vi "Configure Device.vi"(8 "error in":errorcluster, 11 "PPT in":refnum<class "PPT.lvclass">) -> (0 "error out":errorcluster, 3 "PPT out":refnum<class "PPT.lvclass">, 4 "SP":dbl, 5 "Settable?":bool)   [LabVIEW 2018, in "PPT Library.lvlib" / "PPT.lvclass"]
uses:
  PPT.lvclass
  reusable/Session APIs/Serial/Serial Session.lvclass
  <vilib>/Utility/config.llb/NI_LVConfig.lvlib
  <vilib>/Utility/config.llb/Read Key (String).vi
  <vilib>/Utility/config.llb/Read Key (U32).vi
  reusable/Session APIs/File Access/Config Data/Config Data.lvclass
  reusable/Session APIs/Session Log/System Log.lvclass
  Configurable Device/Configurable Device.lvclass
  <vilib>/ErrorRing/Error Ring.xnode
  C:/Program Files (x86)/National Instruments/LabVIEW 2018/user.lib/_Session Fwk/Session - Root.lvclass
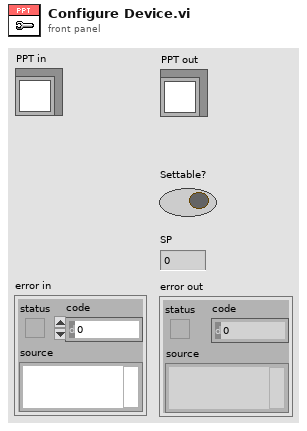
[diagram p1: front panel]
types:
  T1 = enum16{"atm", "bar", "cmwc", "ftwc", "inhg", "inwc", "kgcm", "kpa", "mbar", "mmhg", "mpa", "mwc", "psi", "user", "lcom", "pfs"}
  T2 = typedef "Serial Session.lvclass/Session Handle.ctl" = refnum<data-value>
  T3 = typedef "Config Data.lvclass/Config Session.ctl" = refnum<data-value>
  T4 = typedef "NI_LVConfig.lvlib/Config Data RefNum.ctl" = refnum<k1>
  T5 = typedef "Session - Root.lvclass/Session Handle.ctl" = refnum<data-value>
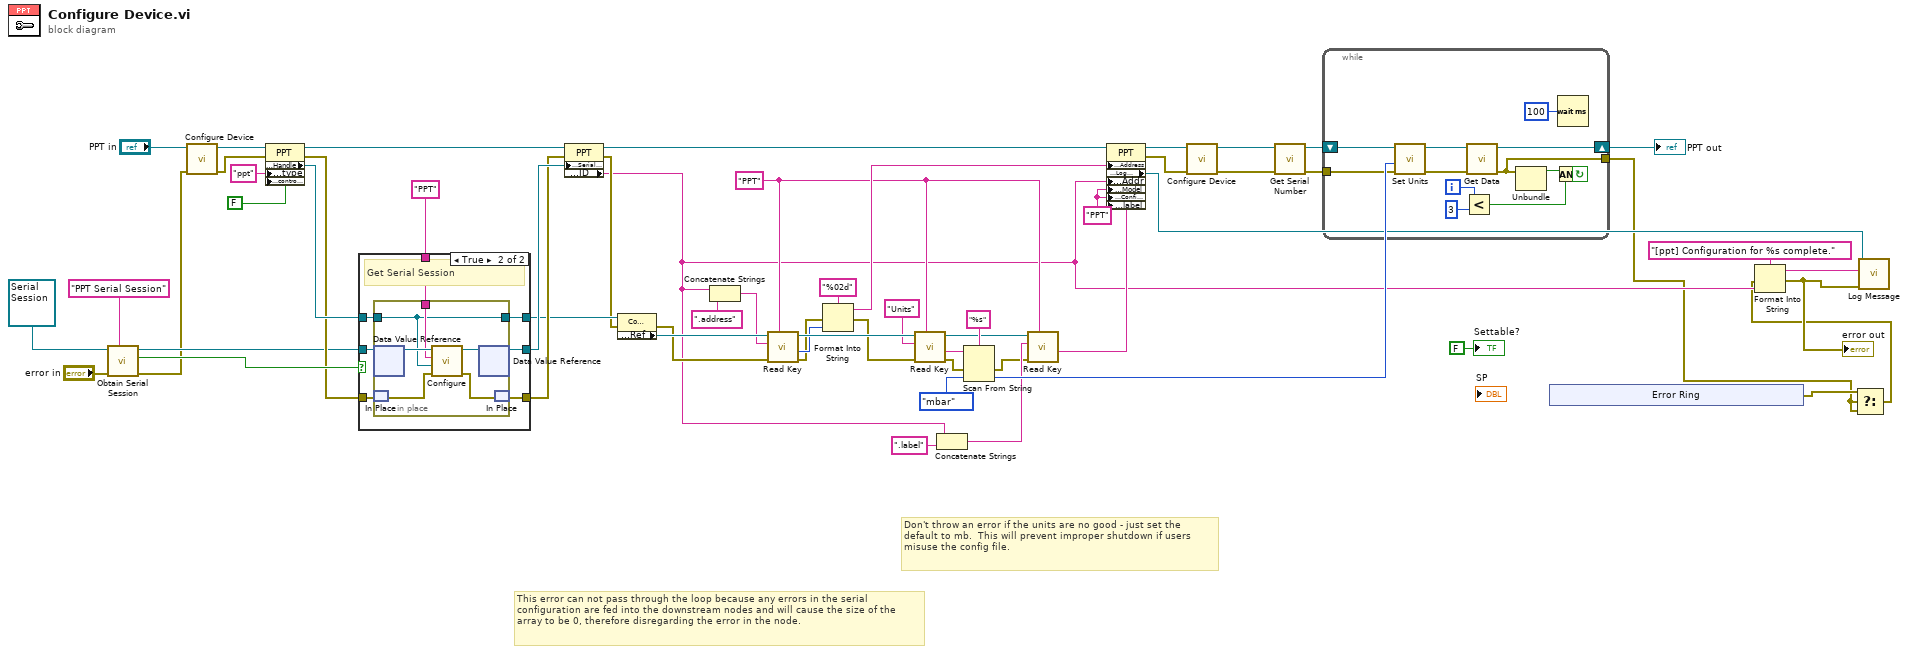
[diagram p0: block diagram]
diagram:
  w5 = "PPT" ("Model")
  w14 = "PPT" ("section")
  # "This error can not pass through the loop because any errors in the serial configuration are fed into the downstream nodes and will cause the size of the array to be 0, therefore disregarding the error in the node."
  # "Don't throw an error if the units are no good - just set the default to mb.  This will prevent improper shutdown if users misuse the config file."
  n1 = call "Obtain Serial Session.vi"("Session Name ()"="PPT Serial Session", "error in"="error in", "Serial Session in"=refnum<class "Serial Session.lvclass"> refnum) -> ("error out"=w19:errorcluster, "created new?"=w61:bool, "hSerial"=w57:T2)  [unwired: 6 in]
  n2 = call-parent "Configure Device.vi"("error in"=w19, "Device in"="PPT in") -> ("error out"=w18:errorcluster, "Device out"=w20:refnum<class "PPT.lvclass">)  [unwired: 6 in, 2 out]
  n3 = property class="PPT"(reference=w20, error in=w18, "Accessors:type"="ppt" ("type"), "Accessors:controller_"=FALSE ("controller_")) -> (reference out=w53:refnum<class "PPT.lvclass">, error out=w59:errorcluster, "Accessors:Handle"=w60:T3)
  n4 = case shown="True" w61 {
    tunnel: w57 -> [w64 w71]
    tunnel: w59 -> [w63 w67]
    tunnel: [w64 w70] -> w52
    tunnel: [w63 w69] -> w51
    tunnel: w60 -> [w62 w68]
    tunnel: [w62 w66] -> w42
    tunnel: "PPT" ("section") -> [_ w65]
    frame False {
    }
    frame True {
      # "Get Serial Session"
      n5 = in-place {
        in-place-border: w68 -> [w72]
        in-place-border: w65 -> [w73]
        in-place-border: [w72] -> w66
        n6 = in-place-dvr #1(w71) -> (w77:refnum<class "Serial Session.lvclass">)  [unwired: 1 out]
        n7 = in-place-match #2(w67) -> (w76:errorcluster)
        n8 = call "Configure.vi"("error in"=w76, "Config Handle"=w72, "section"=w73, "Serial Session in"=w77) -> ("error out"=w75:errorcluster, "Serial Session out"=w74:refnum<class "Serial Session.lvclass">)  [unwired: 6 in]
        n9 = in-place-dvr #1(w74) -> (w70:T2)  [unwired: 1 out]
        n10 = in-place-match #2(w75) -> (w69:errorcluster)
      }
    }
  }
  n11 = property class="PPT"(reference=w53, error in=w51, "Accessors:Serial Session"=w52) -> (reference out=w48:refnum<class "PPT.lvclass">, error out=w41:errorcluster, "Accessors:ID"=w10:string)
  n12 = property class="Config Data"(reference=w42, error in=w41) -> (error out=w29:errorcluster, "Accessors:Ref"=w40:T4)  [unwired: 1 out]
  n13 = Concatenate Strings(w10, ".address" ("string")) -> (w13:string)
  n14 = call-poly <vilib>:"Read Key.vi"("section"=w14, "error in (no error)"=w29, "key"=w13, "refnum"=w40) -> ("error out"=w28:errorcluster, "value"=w38:u32, "refnum out"=w50:T4)  [unwired: 4 in, 1 out]
  n15 = Format Into String(format string="%02d", error in=w28, w38) -> (resulting string=w47:string, error out=w27:errorcluster)  [unwired: 1 in]
  n16 = call-poly <vilib>:"Read Key.vi"("section"=w14, "error in (no error)"=w27, "key"="Units", "refnum"=w50) -> ("error out"=w33:errorcluster, "value"=w46:string, "refnum out"=w15:T4)  [unwired: 4 in, 1 out]
  n17 = Concatenate Strings(w10, ".label" ("string")) -> (w16:string)
  n18 = Scan From String(format string="%s", input string=w46, error in=w33, default 1=T1."mbar" ("units")) -> (error out=w11:errorcluster, output 1=w43:T1)  [unwired: 1 in, 2 out]
  n19 = call-poly <vilib>:"Read Key.vi"("section"=w14, "error in (no error)"=w11, "key"=w16, "refnum"=w15) -> ("value"=w12:string)  [unwired: 4 in, 3 out]
  n20 = property class="PPT"(reference=w48, "Accessors:Address"=w47, "Accessors:Addr"=w10, "Accessors:Model"=w5, "Accessors:Config Section"=w5, "Accessors:label"=w12) -> (reference out=w4:refnum<class "PPT.lvclass">, error out=w2:errorcluster, "Accessors:Log Session"=w36:T5)  [unwired: 1 in]
  n21 = call-parent "Configure Device.vi"("error in"=w2, "Device in"=w4) -> ("error out"=w1:errorcluster, "Device out"=w3:refnum<class "PPT.lvclass">)  [unwired: 6 in, 2 out]
  n22 = call "Get Serial Number.vi"("error in"=w1, "PPT in"=w3) -> ("error out"=w24:errorcluster, "PPT out"=w25:refnum<class "PPT.lvclass">)  [unwired: 7 in, 1 out]
  n23 = call "Set Units.vi"("error in"=w24, "units"=w43, "PPT in"=w25) -> ("error out"=w30:errorcluster, "PPT out"=w32:refnum<class "PPT.lvclass">)  [unwired: 7 in]
  n24 = while {
    shift-right: [w86] -> w31
    shift-left: w32 -> [w87]
    tunnel: [w80] -> w7
    tunnel: w30 -> [w79]
    i -> [w84]
    stop <- w81 continue-if-true
    n25 = Less?(x=w84, y=3) -> (x < y?=w82:bool)
    n26 = call-dynamic "Get Data.vi"("error in"=w79, "PPT in"=w87) -> ("error out"=w80:errorcluster, "PPT out"=w86:refnum<class "PPT.lvclass">)  [unwired: 7 in, 1 out]
    n27 = Unbundle(w80) -> ("status"=w85:bool)  [unwired: 2 out]
    n28 = And(x=w85, y=w82) -> (x .and. y?=w81:bool)
    n29 = Wait (ms)(milliseconds to wait=u32 100) -> ()  [unwired: 1 out]
  }
  "PPT out" <- w31
  n30 = xnode "Error Ring"() -> ("error out"=w8:errorcluster)
  n31 = Select(t=w8, s=w7, f=w7) -> (s? t:f=w6:errorcluster)
  n32 = Format Into String(format string="[ppt] Configuration for %s complete.", error in=w6, w10) -> (resulting string=w34:string, error out=w9:errorcluster)  [unwired: 1 in]
  "error out" <- w9
  n33 = call "Log Message.vi"("error in"=w9, "MSG In"=w34, "session in"=w36) -> ()  [unwired: 7 in, 2 out]
  "Settable?" <- FALSE ("Settable?")
